vi "LvHostsEdit4cRIO_SUB_HostInfo_FromString.vi"(9 "HostInfo[]":T1[](array[typedef])=[{"enable"=TRUE, "IP"="127.0.0.1", "Hostname"="localhost", "Alias"="", "Comment"=""}], 11 "hosts data":string) -> (1 "hosts data out":string, 3 "HostInfo[] out":T1[](array[typedef])=[{"enable"=TRUE, "IP"="127.0.0.1", "Hostname"="localhost", "Alias"="", "Comment"=""}])   [LabVIEW 2014]
uses:
  LvHostsEdit4cRIO_Rsc_HostInfo_Typedef.ctl
panel:
  # "hosts ファイルから読み込んだ文字列を HostInfo形式に読み込み、または逆に書き込み"
  # "純粋に Linux/Unix用(または、または、Windows)のHostsファイルだと、\nファイル先頭にコメントがたくさん入っていたりするが、\ncRIO用のデフォルトHostsファイルは、localhostの定義しかないので、\n単なるタブ区切りとして、読み書きする。"
  # "127.0.0.1\tlocalhost.localdomain\t\tlocalhost"
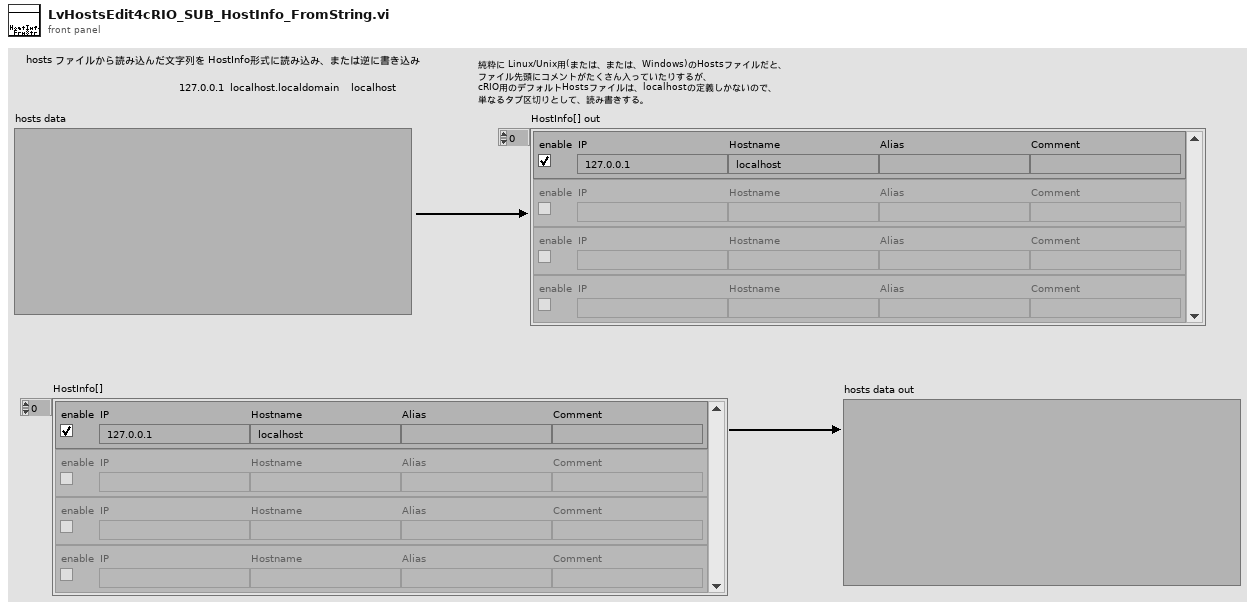
[diagram p1: front panel]
types:
  T1 = typedef "LvHostsEdit4cRIO_Rsc_HostInfo_Typedef.ctl" = cluster{"enable":bool, "IP":string, "Hostname":string, "Alias":string, "Comment":string}
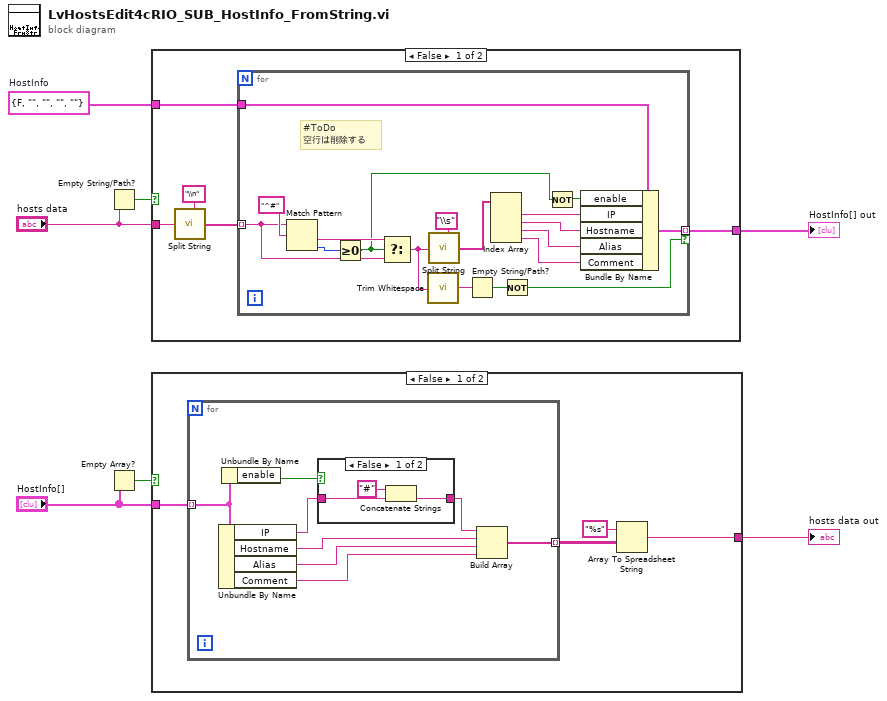
[diagram p0: block diagram]
diagram:
  w6 = T1 {"enable"=FALSE, "IP"="", "Hostname"="", "Alias"="", "Comment"=""}  # HostInfo
  n1 = Empty String/Path?(string/path="hosts data") -> (empty?=w5:bool)
  n2 = Empty Array?(array="HostInfo[]") -> (empty?=w2:bool)
  n3 = case shown="FALSE" w5 {
    tunnel: "hosts data" -> [w12 _]
    tunnel: [w9 _] -> w7
    tunnel: w6 -> [w8 _]
    frame False {
      n4 = call <vilib>:"Split String.vi"("Split Pattern"="\\n", "Input String"=w12) -> ("Split String"=w10:string[])  [unwired: 5 in]
      n5 = for {
        tunnel: w10 -> [w27] mode=indexing
        tunnel: w8 -> [w23]
        tunnel: [w17] -> w9 mode=indexing if=w13
        # "#ToDo\n空行は削除する"
        n6 = Match Pattern(string=w27, regular expression="^#" ("文字列")) -> (after substring=w28:string, offset past match=w29:i32)  [unwired: 1 in, 2 out]
        n7 = Greater Or Equal To 0?(x=w29) -> (x >= 0?=w26:bool)
        n8 = Select(t=w28, s=w26, f=w27) -> (s? t:f=w16:string)
        n9 = call <vilib>:"Trim Whitespace.vi"("string"=w16) -> ("trimmed string"=w15:string)  [unwired: 1 in]
        n10 = call <vilib>:"Split String.vi"("Split Pattern"="\\s", "Input String"=w16) -> ("Split String"=w24:string[])  [unwired: 5 in]
        n11 = Empty String/Path?(string/path=w15) -> (empty?=w14:bool)
        n12 = Index Array(array=w24) -> (element #1=w21:string, element #2=w20:string, element #3=w19:string, element #4=w18:string)  [unwired: 4 in]
        n13 = Not(x=w14) -> (.not. x?=w13:bool)
        n14 = Not(x=w26) -> (.not. x?=w22:bool)
        n15 = Bundle By Name(cluster=w23, "enable"=w22, "IP"=w21, "Hostname"=w20, "Alias"=w19, "Comment"=w18) -> (w17:T1)
      }
    }
    frame True {
    }
  }
  "HostInfo[] out" <- w7
  n16 = case shown="FALSE" w2 {
    tunnel: "HostInfo[]" -> [w34 _]
    tunnel: [w31 _] -> w3
    frame False {
      n17 = for {
        tunnel: w34 -> [w42] mode=indexing
        tunnel: [w35] -> w33 mode=indexing
        n18 = Unbundle By Name(w42) -> ("IP"=w37:string, "Hostname"=w41:string, "Alias"=w40:string, "Comment"=w39:string)
        n19 = Unbundle By Name(w42) -> ("enable"=w38:bool)
        n20 = case shown="FALSE" w38 {
          tunnel: w37 -> [w45 w46]
          tunnel: [w44 w46] -> w36
          frame False {
            n21 = Concatenate Strings("#" ("文字列"), w45) -> (w44:string)
          }
          frame True {
          }
        }
        n22 = Build Array(w36, w41, w40, w39) -> (w35:string[])
      }
      n23 = Array To Spreadsheet String(array=w33, 3:"%s" ("形式文字列")) -> (spreadsheet string=w31:string)  [unwired: 1 in]
    }
    frame True {
    }
  }
  "hosts data out" <- w3
